vi "Export File.vi"() -> ()   [LabVIEW 2011]
panel:
  in  "ppView":variant
  in  "ppDoc":variant
  in  "PLTS.IPLTSview":refnum<k7>
  in  "PLTS.IPLTSDoc":refnum<k7>
  in  "Path":path=path "D:/TX3.s4p"
  in  "Analysis Type":T1(ring)
  in  "PLTS.IPLTSApplication":refnum<k7>
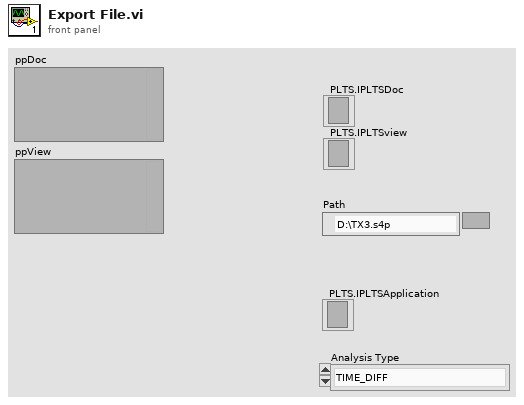
[diagram p1: front panel]
types:
  T1 = enum16{"TIME_DIFF", "TIME_SNGL", "FREQ_BAL", "FRE_SNGL", "EYE_DIFF", "EYE_SNGL"}
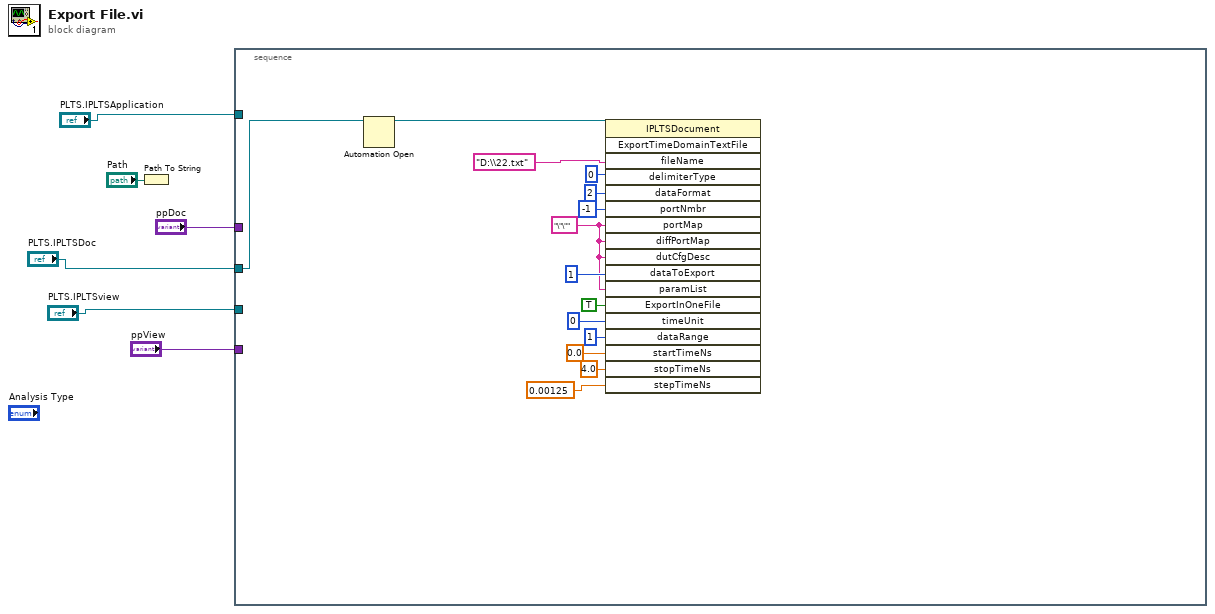
[diagram p0: block diagram]
diagram:
  n1 = Path To String(path="Path") -> ()  [unwired: 1 out]
  n2 = stacked-sequence {
    tunnel: "PLTS.IPLTSApplication" -> [_]
    tunnel: "PLTS.IPLTSDoc" -> [w20]
    tunnel: "PLTS.IPLTSview" -> [_]
    tunnel: "ppDoc" -> [_]
    tunnel: "ppView" -> [_]
    frame #0 {
      w7 = "\"\"" ("portMap")
      n3 = Automation Open(Automation Refnum=w20) -> (Automation Refnum=w19:refnum<k7>)  [unwired: 3 in, 1 out]
      n4 = invoke class="IPLTSDocument" method="ExportTimeDomainTextFile"(reference=w19, "fileName"="D:\\22.txt", "delimiterType"=i16 0, "dataFormat"=i16 2, "portNmbr"=i16 -1, "portMap"=w7, "diffPortMap"=w7, "dutCfgDesc"=w7, "dataToExport"=i16 1, "paramList"=w7, "ExportInOneFile"=TRUE, "timeUnit"=i16 0, "dataRange"=i16 1, "startTimeNs"=0.0, "stopTimeNs"=4.0, "stepTimeNs"=0.00125) -> ()  [unwired: 2 in, 18 out]
    }
  }
